vi "CA Pressure.vi"(2 "Therapy Parameters":T1 {"Aamplitude (mV)" min=50 max=1000 format="%.2f"; "Cycles (s)" format="%.3f"; "Theraputic Freq (MHz)" format="%.3f"}, 3 "Cal Date":enum16{"April 2007", "Jan 2008"}(ring)=enum."Jan 2008") -> (0 "p (MPa)":dbl)   [LabVIEW 2022 SP3]
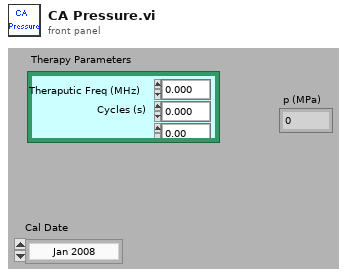
[diagram p1: front panel]
types:
  T1 = cluster{"Theraputic Freq (MHz)":sgl, "Cycles (s)":sgl, "Aamplitude (mV)":sgl, "Lines Before":u16, "Lines After":u16}
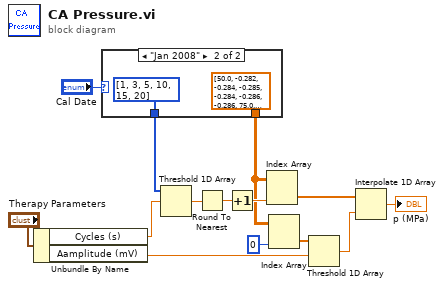
[diagram p0: block diagram]
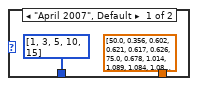
[diagram p2: hidden frame]
diagram:
  n1 = Unbundle By Name("Therapy Parameters") -> ("Cycles (s)"=w5:sgl, "Aamplitude (mV)"=w4:sgl)
  n2 = case shown="\"Jan 2008\"" "Cal Date" {
    tunnel: [dbl[][] [[50.0, 0.356, 0.602, 0.621, 0.617, 0.626], [75.0, 0.678, 1.014, 1.089, 1.084, 1.086], [100.0, 1.04, 1.581, 1.678, 1.699, 1.708], [125.0, 1.419, 2.234, 2.357, 2.362, 2.372], [150.0, 1.657, 2.78, 2.879, 2.92, 2.926], [175.0, 2.019, 3.228, 3.392, 3.436, 3.456], [200.0, 2.352, 3.663, 3.873, 3.922, 3.921], [225.0, 2.65, 3.991, 4.22, 4.283, 4.285], [250.0, 2.95, 4.323, 4.58, 4.663, 4.666], [275.0, 3.203, 4.581, 4.87, 4.958, 4.963], [300.0, 3.455, 4.83, 5.128, 5.202, 5.2], [325.0, 3.705, 5.05, 5.36, 5.41, 5.424], [350.0, 3.958, 5.227, 5.549, 5.639, 5.619], [375.0, 4.16, 5.398, 5.716, 5.806, 5.791], [400.0, 4.359, 5.523, 5.858, 5.94, 5.973], [425.0, 4.536, 5.657, 5.945, 6.081, 6.034], [450.0, 4.711, 5.751, 6.076, 6.181, 6.16], [475.0, 4.859, 5.851, 6.164, 6.267, 6.264], [500.0, 4.988, 5.913, 6.264, 6.355, 6.358]] ("pressures") dbl[][] [[50.0, -0.282, -0.284, -0.285, -0.284, -0.286, -0.286], [75.0, -0.585, -0.776, -0.783, -0.779, -0.782, -0.786], [100.0, -0.814, -1.079, -1.089, -1.091, -1.099, -1.094], [125.0, -1.046, -1.457, -1.461, -1.46, -1.465, -1.471], [150.0, -1.265, -1.718, -1.72, -1.705, -1.721, -1.719], [175.0, -1.439, -2.097, -2.111, -2.097, -2.113, -2.12], [200.0, -1.648, -2.439, -2.468, -2.448, -2.472, -2.47], [225.0, -1.841, -2.771, -2.807, -2.802, -2.831, -2.821], [250.0, -2.06, -3.035, -3.101, -3.099, -3.122, -3.119], [275.0, -2.284, -3.3, -3.4, -3.39, -3.437, -3.425], [300.0, -2.487, -3.539, -3.698, -3.663, -3.718, -3.711], [325.0, -2.684, -3.757, -3.911, -3.928, -3.971, -3.97], [350.0, -2.866, -3.962, -4.168, -4.191, -4.223, -4.22], [375.0, -3.026, -4.148, -4.38, -4.419, -4.447, -4.447], [400.0, -3.159, -4.322, -4.559, -4.603, -4.625, -4.631], [425.0, -3.333, -4.494, -4.721, -4.751, -4.8, -4.8], [450.0, -3.472, -4.596, -4.869, -4.927, -4.971, -4.964], [475.0, -3.608, -4.714, -5.03, -5.067, -5.126, -5.116], [500.0, -3.748, -4.809, -5.156, -5.232, -5.285, -5.246], [525.0, -3.82, -4.894, -5.279, -5.317, -5.376, -5.356], [550.0, -3.942, -4.974, -5.348, -5.43, -5.489, -5.471], [575.0, -4.029, -5.043, -5.457, -5.507, -5.543, -5.54], [600.0, -4.113, -5.133, -5.54, -5.596, -5.634, -5.621], [625.0, -4.194, -5.199, -5.599, -5.667, -5.712, -5.692], [650.0, -4.27, -5.263, -5.668, -5.726, -5.757, -5.765], [675.0, -4.302, -5.294, -5.716, -5.811, -5.856, -5.829], [700.0, -4.337, -5.354, -5.729, -5.822, -5.85, -5.893]] ("first row")] -> w2
    tunnel: [i32[] [1, 3, 5, 10, 15] ("pressures") i32[] [1, 3, 5, 10, 15, 20] ("pressures")] -> w1
    frame "April 2007", Default {
    }
    frame "Jan 2008" {
    }
  }
  n3 = Threshold 1D Array(2:w5, 3:w1) -> (0:w13:dbl)  [unwired: 1 out]
  n4 = Round To Nearest(number=w13) -> (nearest integer value=w12:dbl)
  n5 = Increment(x=w12) -> (x+1=w11:dbl)
  n6 = Index Array(array=w2, index (col)=w11) -> (element=w9:dbl[])  [unwired: 1 in]
  n7 = Index Array(array=w2, index (col)=0 ("disabled index (col)")) -> (element=w10:dbl[])  [unwired: 1 in]
  n8 = Threshold 1D Array(2:w4, 3:w10) -> (0:w8:dbl)  [unwired: 1 out]
  n9 = Interpolate 1D Array(1:w8, 2:w9) -> (0:→"p (MPa)":dbl)
